vi "1A Read Sensor Data.vi"() -> ()   [LabVIEW 2011]
uses:
  2-RIO/2 Typedefs/indicator LED.ctl
  2-RIO/2 Globals/2 Global.vi
panel:
  out "read buffer":string
  out "incoming sentence":string
  in  "stop":bool
  out "Current Status":enum16{"Waiting", "Reading", "Time Out!"}(ring)
  in  "VISA resource name":refnum<visa-resource-name>="COM1"
  in  "error in (no error)":errorcluster
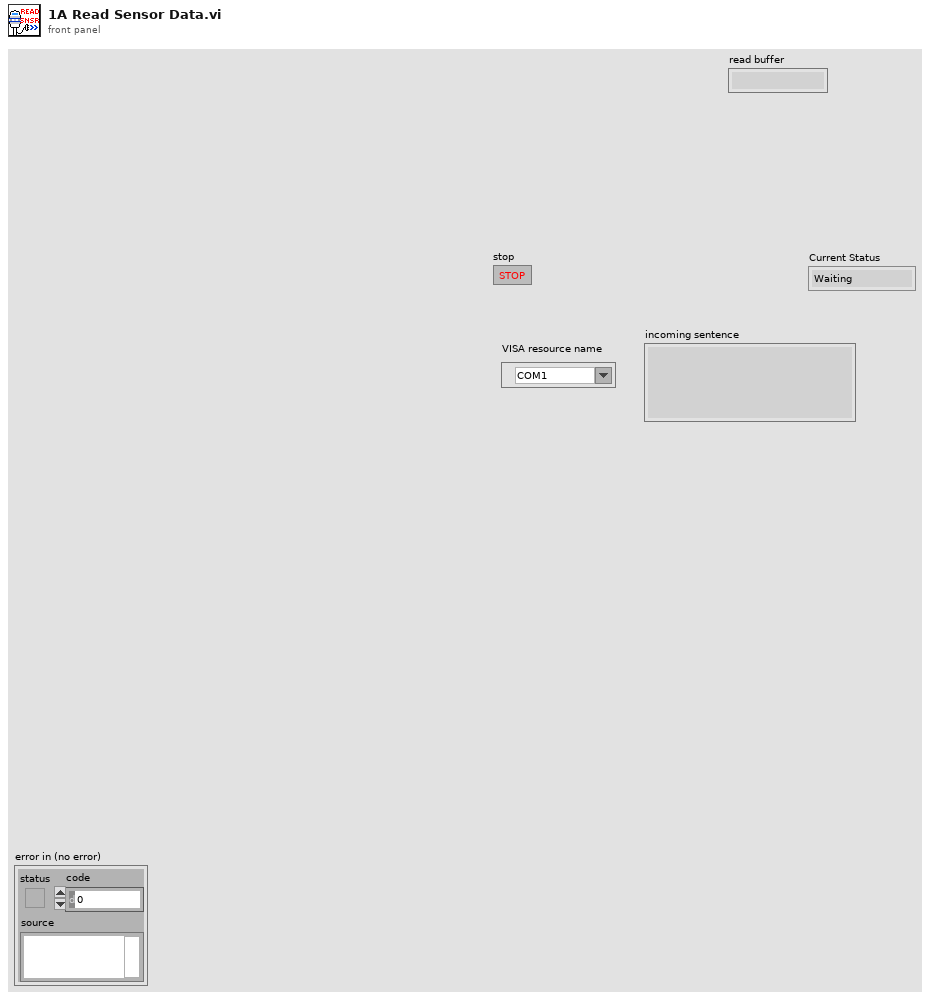
[diagram p1: front panel]
types:
  T1 = typedef "indicator LED.ctl" = bool
  T2 = typedef "generalized sensor status.ctl" = cluster{"Sensor Connected":T1, "Sensor Initialized":T1, "Sensor OK":T1, "Latest Error String":string}
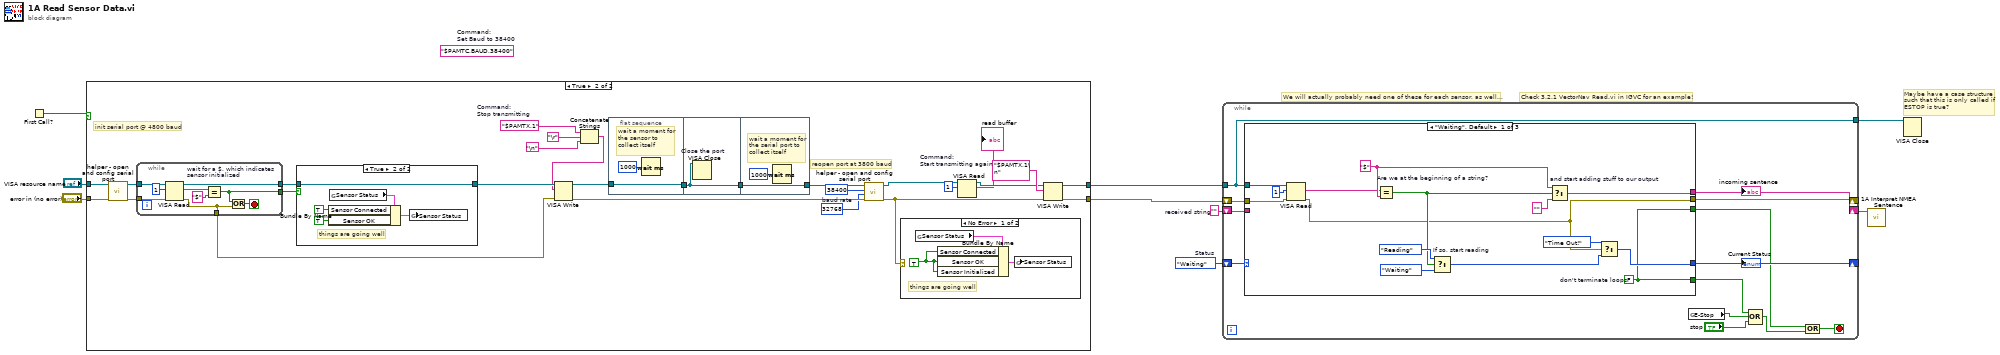
[diagram p0: block diagram]
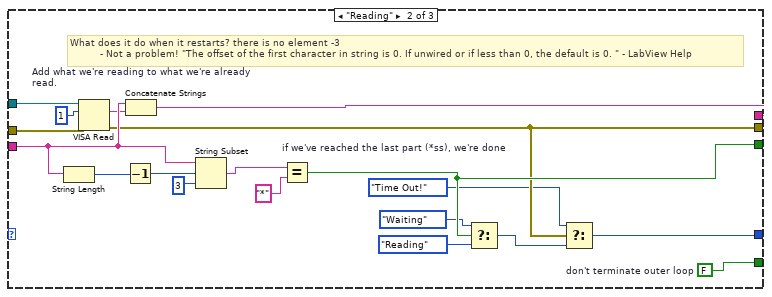
[diagram p2: hidden frame]
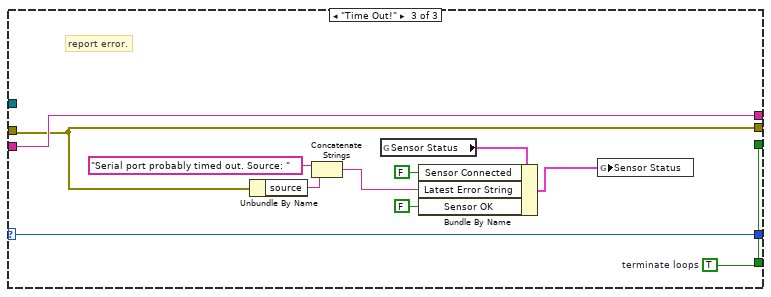
[diagram p3: hidden frame]
diagram:
  (unwired) "$PAMTC,BAUD,38400"  # Command:  Set Baud to 38400
  w1 = enum16{"Waiting", "Reading", "Time Out!"}."Waiting"  # Status
  w3 = ""  # received string
  # "Maybe have a case structure such that this is only called if ESTOP is true?"
  # "Check 3.2.1 VectorNav Read.vi in IGVC for an example!"
  # "We will actually probably need one of these for each sensor, as well..."
  n1 = First Call?() -> (First Call?: T/F=w7:bool)
  n2 = case shown="True" w7 {
    tunnel: [w11 w29] -> w6
    tunnel: [w10 w23] -> w8
    tunnel: "VISA resource name" -> [w11 w28]
    tunnel: "error in (no error)" -> [w10 w27]
    frame False {
    }
    frame True {
      w30 = "$PAMTX,1\n"  # Command: Start transmitting again
      w34 = u32 38400  # baud rate
      w15 = "$PAMTX,1"  # Command:  Stop transmitting
      # "reopen port at 3800 baud"
      # "init serial port @ 4800 baud"
      n3 = call "helper - open and config serial port.vi"("error in (no error)"=w27, "VISA Refnum in"=w28) -> ("error out"=w26:errorcluster, "VISA Refnum out"=w31:refnum<visa-resource-name>)  [unwired: 8 in]
      n4 = while {
        tunnel: w31 -> [w52]
        tunnel: [w49] -> w38
        tunnel: [w51] -> w36
        tunnel: w26 -> [w50]
        tunnel: [w47] -> w25
        stop <- w48 stop-if-true
        n5 = VISA Read(VISA resource name=w52, byte count=u32 1, error in (no error)=w50) -> (VISA resource name out=w51:refnum<visa-resource-name>, read buffer=w54:string, error out=w47:errorcluster)  [unwired: 1 out]
        n6 = Equal? "wait for a $, which indicates\nsensor initialized"(x=w54, y="$" ("x")) -> (x = y?=w49:bool)
        n7 = Or(x=w49, y=w47) -> (x .or. y?=w48:bool)
      }
      n8 = case shown="True" w38 {
        tunnel: [w56 w57] -> w37
        tunnel: w36 -> [w56 w57]
        frame False {
        }
        frame True {
          # "things are going well"
          n9 = global read "2 Global.vi" "Sensor Status"() -> (w60:T2)
          n10 = Bundle By Name(cluster=w60, "Sensor Connected"=T1 TRUE, "Sensor OK"=T1 TRUE) -> (w61:T2)
          n11 = global write "2 Global.vi" "Sensor Status"(w61) -> ()
        }
      }
      n12 = Concatenate Strings(w15, "\r" ("Carriage Return Constant"), "\n") -> (w14:string)
      n13 = VISA Write(VISA resource name=w37, write buffer=w14, error in (no error)=w25) -> (VISA resource name out=w35:refnum<visa-resource-name>, error out=w33:errorcluster)  [unwired: 1 out]
      n14 = flat-sequence {
        tunnel: w35 -> [w42]
        tunnel: [w42] -> w22
        tunnel: w22 -> [w44]
        tunnel: [w44] -> w17
        tunnel: [w46] -> w32
        tunnel: w17 -> [w46]
        frame #0 {
          # "wait a moment for the sensor to collect itself"
          n15 = Wait (ms)(milliseconds to wait=u32 1000) -> ()  [unwired: 1 out]
        }
        frame #1 {
          n16 = VISA Close "Close the port"(VISA resource name=w44) -> ()  [unwired: 1 in, 1 out]
        }
        frame #2 {
          # "wait a moment for the serial port to collect itself"
          n17 = Wait (ms)(milliseconds to wait=u32 1000) -> ()  [unwired: 1 out]
        }
      }
      n18 = call "helper - open and config serial port.vi"("error in (no error)"=w33, "Input\nbuffer size"=u32 32768 ("Input\nbuffer size"), "baud rate"=w34, "VISA Refnum in"=w32) -> ("error out"=w24:errorcluster, "VISA Refnum out"=w21:refnum<visa-resource-name>)  [unwired: 6 in]
      n19 = case shown="No Error" w24 {
        frame No Error {
          w39 = T1 TRUE ("Sensor OK")
          # "things are going well"
          n20 = global read "2 Global.vi" "Sensor Status"() -> (w40:T2)
          n21 = Bundle By Name(cluster=w40, "Sensor Connected"=w39, "Sensor OK"=w39, "Sensor Initialized"=w39) -> (w41:T2)
          n22 = global write "2 Global.vi" "Sensor Status"(w41) -> ()
        }
        frame Error {
        }
      }
      n23 = VISA Read(VISA resource name=w21, byte count=u32 1) -> (VISA resource name out=w20:refnum<visa-resource-name>, read buffer=→"read buffer":string)  [unwired: 1 in, 2 out]
      n24 = VISA Write(VISA resource name=w20, write buffer=w30, error in (no error)=w24) -> (VISA resource name out=w29:refnum<visa-resource-name>, error out=w23:errorcluster)  [unwired: 1 out]
    }
  }
  n25 = while {
    shift-right: [w62] -> w2
    shift-left: w3 -> [w74]
    shift-right: [w71] -> _
    shift-left: w1 -> [w73]
    tunnel: w6 -> [w69]
    tunnel: [w69] -> w9
    shift-right: [w67] -> _
    shift-left: w8 -> [w68]
    stop <- w72 stop-if-true
    n26 = case shown="\"Waiting\", Default" w73 {
      selector: w73 -> [_ _ w119]
      tunnel: w74 -> [_ w102 w118]
      tunnel: [w85 w108 w118] -> w62
      tunnel: [w79 w93 w119] -> w71
      tunnel: [w75 w99 w109] -> w70
      tunnel: w69 -> [w82 w97 _]
      tunnel: w68 -> [w80 w95 w117]
      tunnel: [w77 w94 w117] -> w67
      tunnel: [w75 w90 w109] -> w63
      frame "Waiting", Default {
        w75 = FALSE  # don't terminate loops
        w84 = "$" ("x")
        n27 = VISA Read(VISA resource name=w82, byte count=u32 1, error in (no error)=w80) -> (read buffer=w83:string, error out=w77:errorcluster)  [unwired: 2 out]
        n28 = Equal? "Are we at the beginning of a string?"(x=w83, y=w84) -> (x = y?=w86:bool)
        n29 = Select "If so, start reading"(t=enum16{"Waiting", "Reading", "Time Out!"}."Reading", s=w86, f=enum16{"Waiting", "Reading", "Time Out!"}."Waiting" ("Current Status")) -> (s? t:f=w78:enum16{"Waiting", "Reading", "Time Out!"})
        n30 = Select "and start adding stuff to our output"(t=w84, s=w86, f="") -> (s? t:f=w85:string)
        n31 = Select(t=enum16{"Waiting", "Reading", "Time Out!"}."Time Out!", s=w77, f=w78) -> (s? t:f=w79:enum16{"Waiting", "Reading", "Time Out!"})
      }
      frame "Reading" {
        w90 = FALSE  # don't terminate outer loop
        # "What does it do when it restarts? there is no element -3\n          - Not a problem! \"The offset of the first character in string is 0. If unwired or if less than 0, the default is 0. \" - LabView Help"
        n32 = String Length(string=w102) -> (length=w107:i32)
        n33 = VISA Read(VISA resource name=w97, byte count=u32 1, error in (no error)=w95) -> (read buffer=w101:string, error out=w94:errorcluster)  [unwired: 2 out]
        n34 = Decrement(x=w107) -> (x-1=w106:i32)
        n35 = Concatenate Strings "Add what we're reading to what we're already read."(w102, w101) -> (w108:string)
        n36 = String Subset(string=w102, offset (0)=w106, length (rest)=3 ("length (rest)")) -> (substring=w104:string)
        n37 = Equal? "if we've reached the last part (*ss), we're done"(x=w104, y="*") -> (x = y?=w99:bool)
        n38 = Select(t=enum16{"Waiting", "Reading", "Time Out!"}."Waiting", s=w99, f=enum16{"Waiting", "Reading", "Time Out!"}."Reading" ("Status")) -> (s? t:f=w92:enum16{"Waiting", "Reading", "Time Out!"})
        n39 = Select(t=enum16{"Waiting", "Reading", "Time Out!"}."Time Out!", s=w94, f=w92) -> (s? t:f=w93:enum16{"Waiting", "Reading", "Time Out!"})
      }
      frame "Time Out!" {
        w109 = TRUE  # terminate loops
        # "report error."
        n40 = Unbundle By Name(w117) -> ("source"=w111:string)
        n41 = Concatenate Strings("Serial port probably timed out. Source: " ("string"), w111) -> (w112:string)
        n42 = global read "2 Global.vi" "Sensor Status"() -> (w115:T2)
        n43 = Bundle By Name(cluster=w115, "Sensor Connected"=T1 FALSE, "Latest Error String"=w112, "Sensor OK"=T1 FALSE) -> (w114:T2)
        n44 = global write "2 Global.vi" "Sensor Status"(w114) -> ()
      }
    }
    "Current Status" <- w71
    "incoming sentence" <- w62
    n45 = global read "2 Global.vi" "E-Stop"() -> (w65:bool)
    n46 = Compound Arithmetic op=OR(w63, w65, "stop") -> (w64:bool)
    n47 = Compound Arithmetic op=OR(w70, w64) -> (w72:bool)
  }
  n48 = call "1A Interpret NMEA Sentence.vi"("NMEA Sentence"=w2) -> ()  [unwired: 11 in]
  n49 = VISA Close(VISA resource name=w9) -> ()  [unwired: 1 in, 1 out]
